vi "CALC_TRAN_TIME_KBES.vi"(0 "VISA IN":refnum<visa-resource-name>, 1 "Window Width(sec)":dbl, 5 "error in":errorcluster, 7 "Channel":i32) -> (14 "VISA Out":refnum<visa-resource-name>, 19 "error out":errorcluster)   [LabVIEW 2018, in "PNA-X.lvlib"]
doc: "CALCulate<cnum>:TRANsform:TIME:KBESsel <num> \n(Read-Write) Sets the parametric window for the Kaiser Bessel window. \nSee Critical Note \nParameters \n<cnum> Channel number of the measurement. There must be a selected measurement \non that channel. If unspecified, <cnum> is set to 1. \n<num> Window width for Kaiser Bessel in seconds; Choose any number between: \n0.0 and 13.0 \nExamples CALC:TRAN:TIME:KBES 10 \ncalculate2:transform:time:kbessel 13 \nQuery Syntax CALCulate<cnum>:TRANsform:TIME:KBESsel? \nReturn Type Numeric \nDefault 6"
uses:
  PNA-X.lvlib
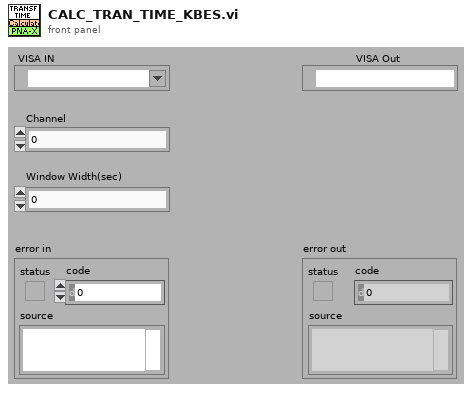
[diagram p1: front panel]
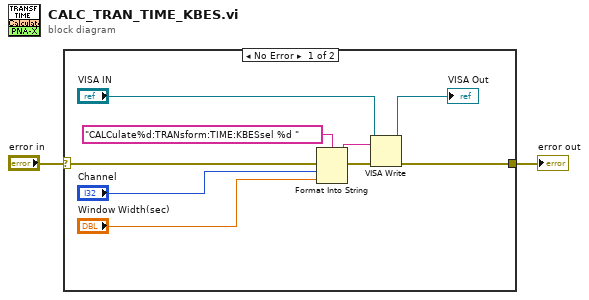
[diagram p0: block diagram]
diagram:
  n1 = case shown="No Error" "error in" {
    selector: "error in" -> [w11 w12]
    tunnel: [w6 w12] -> w1
    frame No Error {
      n2 = Format Into String(format string="CALCulate%d:TRANsform:TIME:KBESsel %d " ("Cmdline"), error in=w11, "Channel", "Window Width(sec)") -> (resulting string=w9:string, error out=w10:errorcluster)  [unwired: 1 in]
      n3 = VISA Write(VISA resource name="VISA IN", write buffer=w9, error in (no error)=w10) -> (VISA resource name out=→"VISA Out":refnum<visa-resource-name>, error out=w6:errorcluster)  [unwired: 1 out]
    }
    frame Error {
    }
  }
  "error out" <- w1
